vi "EXO1.vi"() -> ()   [LabVIEW 2012]
uses:
  <vilib>/FieldPoint/Polymorphic Write.llb/FP Write (Float -IO).vi
  <vilib>/FieldPoint/Polymorphic Read.llb/FP Read (Float Array -IO).vi
  <vilib>/FieldPoint/Polymorphic Read.llb/FP Read (Float -IO).vi
  <vilib>/addons/database/Connection.llb/DB Tools Open Connec (Path).vi
  <instrlib>/Dual Gauge/Dual Gauge.lvlib
  <vilib>/addons/database/NI_Database_API.lvlib
panel:
  out "current time":timestamp
  in  "Table Name (The table that you want to save the data into)":string="exodata"
  in  "Enter Control Mode":bool
  in  "Password":string
  in  "Username":string
  in  "V-20\n(Block)":bool
  out "Flow Speed (L/min)":dbl caption="Pressure" format="%.3e"
  out "LN2 Dewar 2":dbl(slide) scale=0.0..10.0
  out "LN2 Dewar 1":dbl(slide) scale=0.0..10.0
  out "Xenon Cell":dbl(slide) scale=0.0..10.0
  in  "Control Input 2":dbl(slide) scale=0.0..10.0
  in  "Control Input 1":dbl(slide) scale=0.0..10.0
  out "Pressure 3":dbl caption="Pressure" format="%.3e"
  out "Pressure 2":dbl caption="Pressure" format="%.3e"
  out "Pressure 1":dbl caption="Pressure" format="%.3e"
  out "Pressure 4":dbl caption="Pressure" format="%.3e"
  in  "V-10":bool
  in  "Jog":bool
  in  "Reverse / Stop":bool
  in  "Forward / Stop":bool
  in  "Speed Control Knob":dbl(knob) caption="Knob" scale=0.0..10.0 scale format="%^#_6g"
  in  "V-9":bool
  in  "V-19\n(Block)":bool
  in  "V-18\n(Block)":bool
  out "Thermocouple 1":dbl(slide) scale=0.0..100.0
  out "DT 1":dbl(slide) scale=0.0..100.0
  out "PT 1":dbl(slide) scale=0.0..100.0
  in  "V-15":bool
  in  "V-14":bool
  in  "V-7":bool
  in  "R-1":bool
  in  "V-8":bool
  in  "R-2":bool
  in  "V-2":bool
  in  "V-17\n(Proportional)":bool
  in  "V-16\n(Proportional)":bool
  in  "V-6":bool
  in  "V-4":bool
  in  "V-3":bool
  in  "V-5":bool
  in  "stop":bool
  in  "V-13":bool
  in  "V-11":bool
  in  "V-12":bool
  in  "V-1":bool
  # "EXO Front Panel"
  # "Rupture Disc"
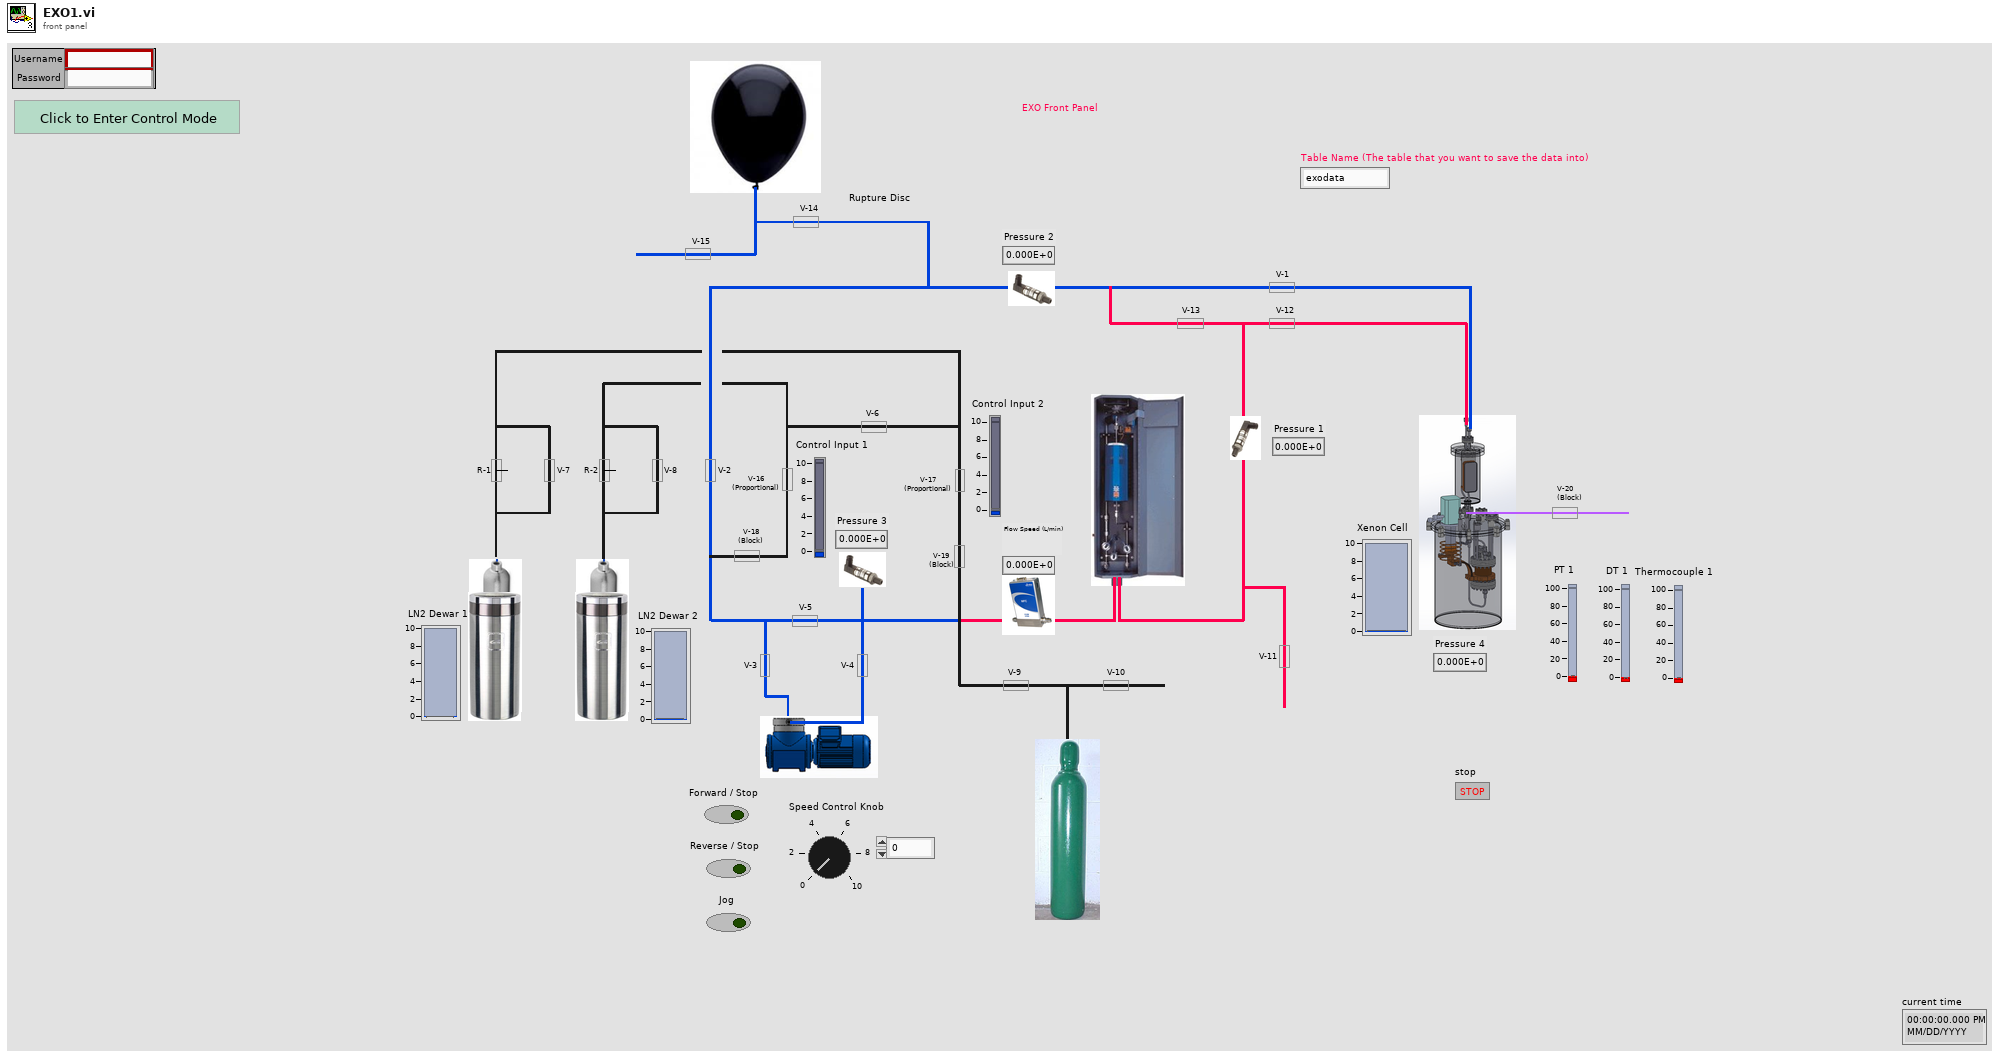
[diagram p1: front panel]
types:
  T1 = cluster{"date/time string":string, "Ch1 [K]":dbl, "Ch2 [K] ":dbl, "value":dbl, "LN2 Dewar 2":dbl, "LN2 Dewar 2":dbl, "LN2 Dewar 2":dbl, "psi":dbl, "psi":dbl, "psi":dbl, dbl, dbl, dbl, dbl, dbl, dbl, dbl, dbl, dbl, dbl, dbl, dbl, dbl, dbl, dbl, dbl}
  T2 = typedef "NI_Database_API.lvlib/Conn ObjectReference.ctl" = refnum<k1>
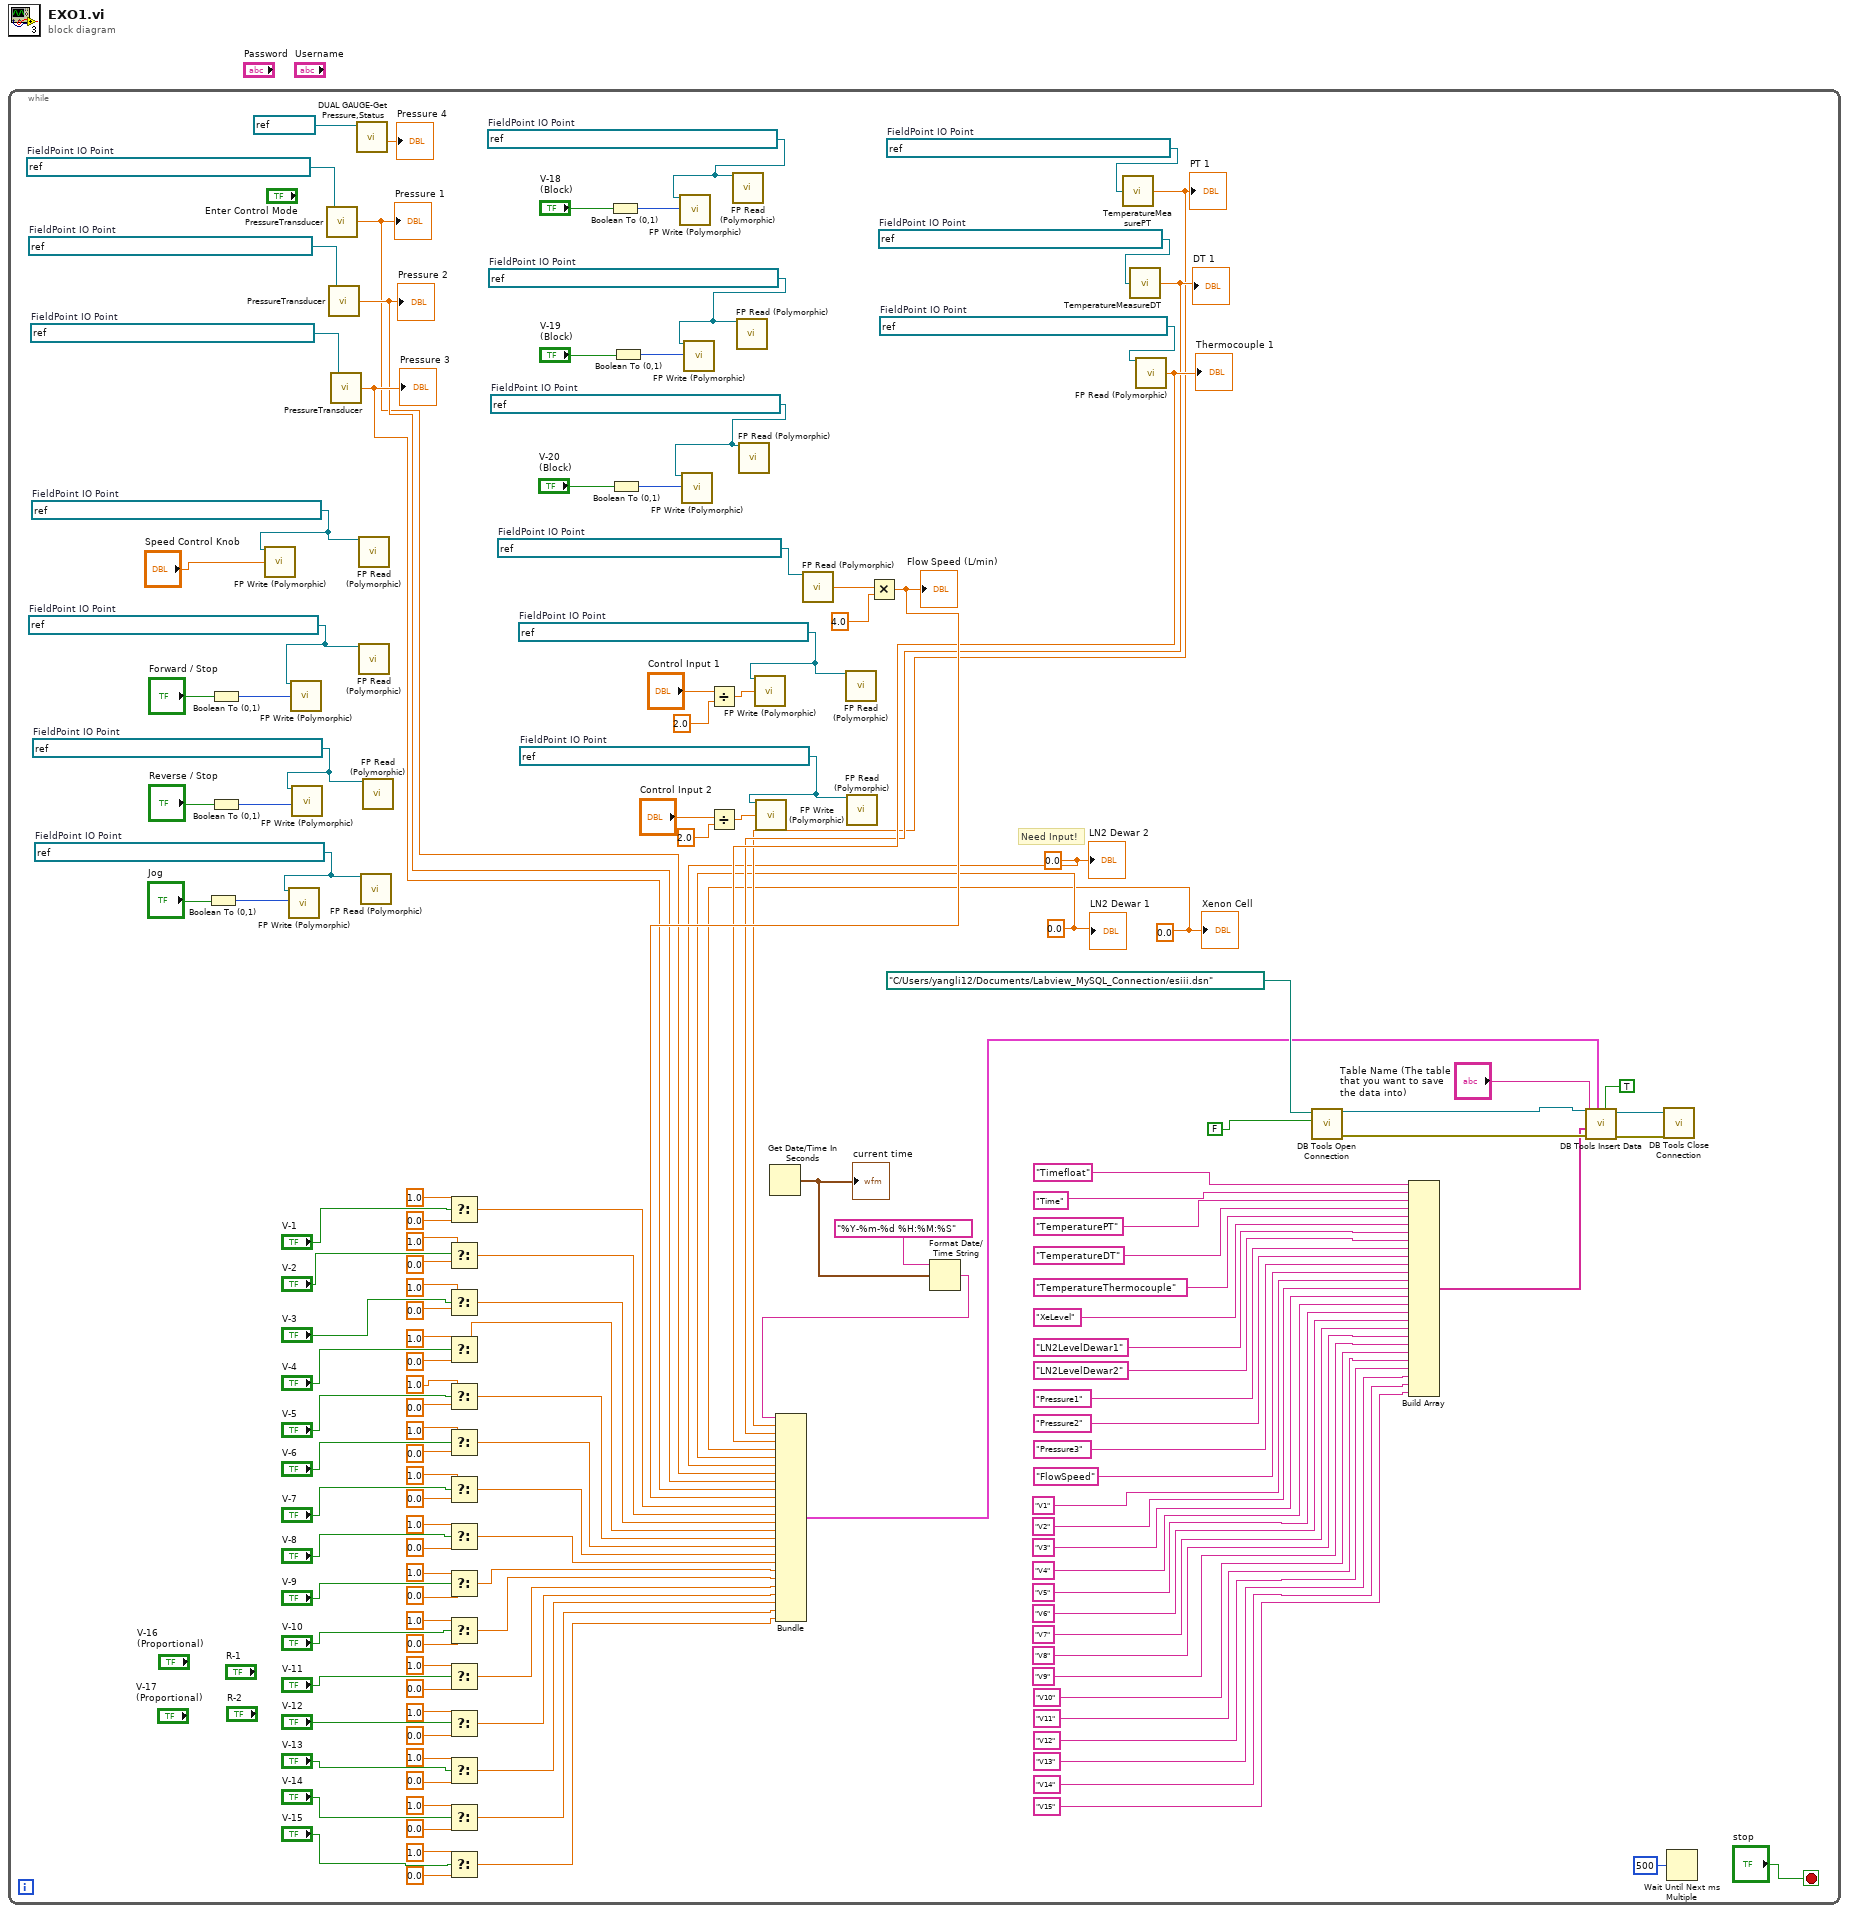
[diagram p0: block diagram]
diagram:
  n1 = while {
    stop <- "stop" stop-if-true
    w3 = 0.0 ("LN2 Dewar 2")
    w4 = 0.0 ("LN2 Dewar 2")
    w5 = 0.0 ("LN2 Dewar 2")
    w113 = refnum<k21> "FieldPoint\\Loomis434\\cFP-DO-401 @4\\Channel 5"  # FieldPoint IO Point
    w117 = refnum<k21> "FieldPoint\\Loomis434\\cFP-AI-112 @5\\Channel 2"  # FieldPoint IO Point
    w118 = refnum<k21> "FieldPoint\\Loomis434\\cFP-DO-401 @4\\Channel 4"  # FieldPoint IO Point
    w121 = refnum<k21> "FieldPoint\\Loomis434\\cFP-DO-401 @4\\Channel 3"  # FieldPoint IO Point
    w130 = refnum<k21> "FieldPoint\\Loomis434\\cFP-AO-210 @2\\Channel 2"  # FieldPoint IO Point
    w131 = refnum<k21> "FieldPoint\\Loomis434\\cFP-AO-210 @2\\Channel 1"  # FieldPoint IO Point
    w132 = refnum<k21> "FieldPoint\\Loomis434\\cFP-AI-100 @6\\Channel 1"  # FieldPoint IO Point
    w133 = refnum<k21> "FieldPoint\\Loomis434\\cFP-AI-100 @6\\Channel 1"  # FieldPoint IO Point
    w134 = refnum<k21> "FieldPoint\\Loomis434\\cFP-AI-100 @6\\Channel 0"  # FieldPoint IO Point
    w136 = refnum<k21> "FieldPoint\\Loomis434\\cFP-TC-120 @3\\Channel 0"  # FieldPoint IO Point
    w137 = refnum<k21> "FieldPoint\\Loomis434\\cFP-AI-112 @5\\Channel 1"  # FieldPoint IO Point
    w138 = refnum<k21> "FieldPoint\\Loomis434\\cFP-AI-112 @5\\Channel 0"  # FieldPoint IO Point
    w141 = refnum<k21> "FieldPoint\\Loomis434\\cFP-DO-401 @4\\Channel 2"  # FieldPoint IO Point
    w143 = refnum<k21> "FieldPoint\\Loomis434\\cFP-DO-401 @4\\Channel 1"  # FieldPoint IO Point
    w146 = refnum<k21> "FieldPoint\\Loomis434\\cFP-DO-401 @4\\Channel 0"  # FieldPoint IO Point
    w149 = refnum<k21> "FieldPoint\\Loomis434\\cFP-AO-210 @2\\Channel 0"  # FieldPoint IO Point
    # "Need Input!"
    n2 = Boolean To (0,1)(Boolean="Jog") -> (0, 1=w142:i16)
    n3 = Boolean To (0,1)(Boolean="Forward / Stop") -> (0, 1=w148:i16)
    n4 = Boolean To (0,1)(Boolean="Reverse / Stop") -> (0, 1=w144:i16)
    n5 = call-poly <vilib>:"FP Write (Polymorphic).vi"("FieldPoint IO Point In"=w149, "value"="Speed Control Knob") -> ()  [unwired: 11 in, 3 out]
    n6 = call-poly <vilib>:"FP Write (Polymorphic).vi"("FieldPoint IO Point In"=w141, "value"=w142) -> ()  [unwired: 11 in, 3 out]
    n7 = call-poly <vilib>:"FP Write (Polymorphic).vi"("FieldPoint IO Point In"=w146, "value"=w148) -> ()  [unwired: 11 in, 3 out]
    n8 = call-poly <vilib>:"FP Write (Polymorphic).vi"("FieldPoint IO Point In"=w143, "value"=w144) -> ()  [unwired: 11 in, 3 out]
    n9 = call "PressureTransducer.vi"("FieldPoint IO Point In"=w134) -> ("psi"=w12:dbl)
    "Pressure 1" <- w12
    n10 = call "PressureTransducer.vi"("FieldPoint IO Point In"=w133) -> ("psi"=w13:dbl)
    "Pressure 2" <- w13
    n11 = call "PressureTransducer.vi"("FieldPoint IO Point In"=w132) -> ("psi"=w14:dbl)
    "Pressure 3" <- w14
    n12 = call <instrlib>:"DUAL GAUGE-Get Pressure,Status.vi"("Referenz in"=refnum<visa-resource-name> "COM7") -> ("Pressure"=→"Pressure 4":dbl)  [unwired: 7 in, 3 out]
    n13 = call-poly <vilib>:"FP Read (Polymorphic).vi"("FieldPoint IO Point In"=w149) -> ()  [unwired: 11 in, 4 out]
    n14 = call-poly <vilib>:"FP Read (Polymorphic).vi"("FieldPoint IO Point In"=w146) -> ()  [unwired: 11 in, 4 out]
    n15 = call-poly <vilib>:"FP Read (Polymorphic).vi"("FieldPoint IO Point In"=w141) -> ()  [unwired: 11 in, 4 out]
    n16 = call-poly <vilib>:"FP Read (Polymorphic).vi"("FieldPoint IO Point In"=w143) -> ()  [unwired: 11 in, 4 out]
    n17 = Select(t=1.0, s="V-1", f=0.0) -> (s? t:f=w75:dbl)
    n18 = Select(t=1.0, s="V-2", f=0.0) -> (s? t:f=w74:dbl)
    n19 = Select(t=1.0, s="V-3", f=0.0) -> (s? t:f=w73:dbl)
    n20 = Select(t=1.0, s="V-4", f=0.0) -> (s? t:f=w72:dbl)
    n21 = Select(t=1.0, s="V-5", f=0.0) -> (s? t:f=w71:dbl)
    n22 = Select(t=1.0, s="V-6", f=0.0) -> (s? t:f=w70:dbl)
    n23 = Select(t=1.0, s="V-7", f=0.0) -> (s? t:f=w69:dbl)
    n24 = Select(t=1.0, s="V-8", f=0.0) -> (s? t:f=w68:dbl)
    n25 = Select(t=1.0, s="V-9", f=0.0) -> (s? t:f=w67:dbl)
    n26 = Select(t=1.0, s="V-10", f=0.0) -> (s? t:f=w66:dbl)
    n27 = Select(t=1.0, s="V-11", f=0.0) -> (s? t:f=w65:dbl)
    n28 = Select(t=1.0, s="V-12", f=0.0) -> (s? t:f=w64:dbl)
    n29 = Select(t=1.0, s="V-13", f=0.0) -> (s? t:f=w63:dbl)
    n30 = Select(t=1.0, s="V-14", f=0.0) -> (s? t:f=w62:dbl)
    n31 = Select(t=1.0, s="V-15", f=0.0) -> (s? t:f=w61:dbl)
    n32 = Boolean To (0,1)(Boolean="V-18\n(Block)") -> (0, 1=w122:i16)
    n33 = Boolean To (0,1)(Boolean="V-20\n(Block)") -> (0, 1=w112:i16)
    n34 = Boolean To (0,1)(Boolean="V-19\n(Block)") -> (0, 1=w119:i16)
    n35 = call-poly <vilib>:"FP Write (Polymorphic).vi"("FieldPoint IO Point In"=w121, "value"=w122) -> ()  [unwired: 11 in, 3 out]
    n36 = call-poly <vilib>:"FP Write (Polymorphic).vi"("FieldPoint IO Point In"=w113, "value"=w112) -> ()  [unwired: 11 in, 3 out]
    n37 = call-poly <vilib>:"FP Write (Polymorphic).vi"("FieldPoint IO Point In"=w118, "value"=w119) -> ()  [unwired: 11 in, 3 out]
    n38 = Divide(x="Control Input 1", y=2.0) -> (x/y=w128:dbl)
    n39 = Divide(x="Control Input 2", y=2.0) -> (x/y=w126:dbl)
    n40 = call-poly <vilib>:"FP Read (Polymorphic).vi"("FieldPoint IO Point In"=w121) -> ()  [unwired: 11 in, 4 out]
    n41 = call-poly <vilib>:"FP Read (Polymorphic).vi"("FieldPoint IO Point In"=w118) -> ()  [unwired: 11 in, 4 out]
    n42 = call-poly <vilib>:"FP Read (Polymorphic).vi"("FieldPoint IO Point In"=w113) -> ()  [unwired: 11 in, 4 out]
    n43 = call-poly <vilib>:"FP Write (Polymorphic).vi"("FieldPoint IO Point In"=w131, "value"=w128) -> ()  [unwired: 11 in, 3 out]
    n44 = call-poly <vilib>:"FP Write (Polymorphic).vi"("FieldPoint IO Point In"=w130, "value"=w126) -> ()  [unwired: 11 in, 3 out]
    n45 = Get Date/Time In Seconds() -> (seconds since 1Jan1904=w8:timestamp)
    "current time" <- w8
    n46 = call-poly <vilib>:"FP Read (Polymorphic).vi"("FieldPoint IO Point In"=w117) -> ("value"=w116:dbl)  [unwired: 11 in, 3 out]
    n47 = call-poly <vilib>:"FP Read (Polymorphic).vi"("FieldPoint IO Point In"=w131) -> ()  [unwired: 11 in, 4 out]
    n48 = call-poly <vilib>:"FP Read (Polymorphic).vi"("FieldPoint IO Point In"=w130) -> ()  [unwired: 11 in, 4 out]
    n49 = Multiply(x=w116, y=4.0) -> (x*y=w15:dbl)
    "Flow Speed (L/min)" <- w15
    n50 = Format Date/Time String(time format string (%c)="%Y-%m-%d %H:%M:%S", seconds (now)=w8) -> (date/time string=w7:string)  [unwired: 1 in]
    n51 = call "TemperatureMeasurePT.vi"("FieldPoint IO Point In"=w138) -> ("Ch1 [K]"=w9:dbl)
    "PT 1" <- w9
    n52 = call "TemperatureMeasureDT.vi"("FieldPoint IO Point In"=w137) -> ("Ch2 [K]"=w10:dbl)
    "DT 1" <- w10
    n53 = call-poly <vilib>:"FP Read (Polymorphic).vi"("FieldPoint IO Point In"=w136) -> ("value"=w11:dbl)  [unwired: 11 in, 3 out]
    "Thermocouple 1" <- w11
    n54 = Bundle("date/time string"=w7, "Ch1 [K]"=w9, "Ch2 [K]"=w10, "value"=w11, "LN2 Dewar 2"=w3, "LN2 Dewar 2"=w4, "LN2 Dewar 2"=w5, "psi"=w12, "psi"=w13, "psi"=w14, w15, w75, w74, w73, w72, w71, w70, w69, w68, w67, w66, w65, w64, w63, w62, w61) -> (w6:T1)  [unwired: 1 in]
    n55 = call-poly <vilib>:"DB Tools Open Connection.vi"("prompt? (F)"=FALSE, "connection information"=path "C:/Users/yangli12/Documents/Labview_MySQL_Connection/esiii.dsn") -> ("error out"=w107:errorcluster, "connection reference"=w108:T2)  [unwired: 6 in]
    n56 = Build Array("Timefloat" ("element"), "Time" ("table"), "TemperaturePT" ("table"), "TemperatureDT" ("table"), "TemperatureThermocouple" ("table"), "XeLevel" ("table"), "LN2LevelDewar1" ("table"), "LN2LevelDewar2" ("table"), "Pressure1" ("table"), "Pressure2" ("table"), "Pressure3" ("table"), "FlowSpeed" ("table"), "V1" ("table"), "V2" ("table"), "V3" ("table"), "V4" ("table"), "V5" ("table"), "V6" ("table"), "V7" ("table"), "V8" ("table"), "V9" ("table"), "V10" ("table"), "V11" ("table"), "V12" ("table"), "V13" ("table"), "V14" ("table"), "V15" ("table")) -> (w103:string[])
    n57 = call <vilib>:"DB Tools Insert Data.vi"("create table? (F)"=TRUE, "data"=w6, "error in (no error)"=w107, "columns"=w103, "table"="Table Name (The table that you want to save the data into)", "connection reference"=w108) -> ("error out"=w100:errorcluster, "connection reference out"=w101:T2)  [unwired: 4 in]
    n58 = call <vilib>:"DB Tools Close Connection.vi"("error in (no error)"=w100, "connection reference"=w101) -> ()  [unwired: 5 in, 1 out]
    n59 = Wait Until Next ms Multiple(millisecond multiple=u32 500) -> ()  [unwired: 1 out]
    "Xenon Cell" <- w3
    "LN2 Dewar 1" <- w4
    "LN2 Dewar 2" <- w5
  }
